vi "GetLoopConditional.vi"(6 "error in":errorcluster, 9 "WhileLoop in":refnum<class "WhileLoop.lvclass">) -> (0 "error out":errorcluster, 3 "WhileLoop out":refnum<class "WhileLoop.lvclass">, 4 "conditional UID":i32)   [LabVIEW 2014, in "WhileLoop.lvclass"]
uses:
  WhileLoop.lvclass
  WhileLoop.lvclass/WhileLoop.ctl
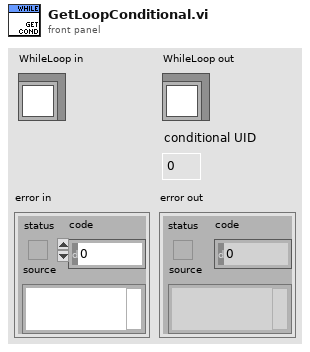
[diagram p1: front panel]
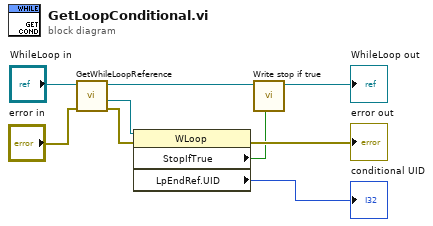
[diagram p0: block diagram]
diagram:
  n1 = call "GetWhileLoopReference.vi"("error in"="error in", "WhileLoop in"="WhileLoop in") -> ("error out"=w6:errorcluster, "reference out"=w7:refnum<vi>, "WhileLoop out"=w3:refnum<class "WhileLoop.lvclass">)  [unwired: 7 in]
  n2 = property class="WLoop"(reference=w7, error in=w6) -> (error out=→"error out":errorcluster, "StopIfTrue"=w2:bool, "LpEndRef.UID"=→"conditional UID":i32)  [unwired: 1 out]
  n3 = call "Write stop if true.vi"("stop if true"=w2, "ForLoop in"=w3) -> ("ForLoop out"=→"WhileLoop out":refnum<class "WhileLoop.lvclass">)  [unwired: 7 in]
